vi "SpreadsheetWrite.vi"() -> ()   [LabVIEW 2014]
uses:
  <vilib>/Utility/file.llb/Write To Spreadsheet File (DBL).vi
panel:
  in  "AM Wave parameters":T1={"Signal Frequency"=50.0, "Amplitude"=5.0, "Modulation Frequency"=0.0}
  in  "Digitalizing Parameters":T2={"Number of Samples"=10.0, "Sampling Frequency"=1000.0}
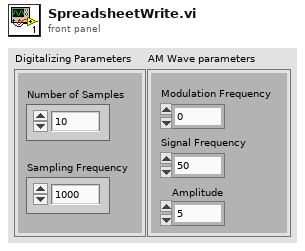
[diagram p1: front panel]
types:
  T1 = cluster{"Signal Frequency":dbl, "Amplitude":dbl, "Modulation Frequency":dbl}
  T2 = cluster{"Number of Samples":dbl, "Sampling Frequency":dbl}
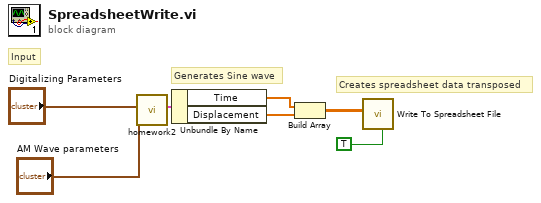
[diagram p0: block diagram]
diagram:
  # "Input"
  # "Generates Sine wave"
  # "Creates spreadsheet data transposed"
  n1 = call "homework2.vi"("AM Wave parameters"="AM Wave parameters", "Digitalizing Parameters"="Digitalizing Parameters") -> ("AM waves"=w5:cluster{"Time":dbl[], "Displacement":dbl[]})  [unwired: 9 in]
  n2 = Unbundle By Name(w5) -> ("Time"=w3:dbl[], "Displacement"=w2:dbl[])
  n3 = Build Array(w3, w2) -> (w1:dbl[][])
  n4 = call-poly <vilib>:"Write To Spreadsheet File.vi"("transpose? (no:F)"=TRUE, "2D data"=w1) -> ()  [unwired: 6 in, 1 out]
